vi "20211029_HW03.vi"() -> ()   [LabVIEW 2019]
panel:
  out "Sum":i32
  in  "N1":i32
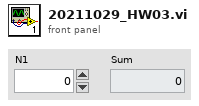
[diagram p1: front panel]
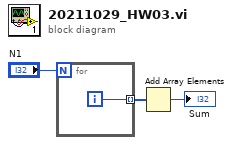
[diagram p0: block diagram]
diagram:
  n1 = for {
    N: "N1" -> [_]
    tunnel: [w4] -> w2 mode=indexing
    i -> [w4]
  }
  n2 = Add Array Elements(numeric array=w2) -> (sum=→"Sum":i32)
